vi "U-I.vi"() -> ()   [LabVIEW 2020]
uses:
  <vilib>/Analysis/baseanly.llb/Mean (DBL).vi
  <vilib>/Analysis/NI_AALBase.lvlib
  <vilib>/Analysis/NI_AALPro.lvlib
panel:
  out "数据":dbl[][](array[numeric])
  out "待测电阻值":dbl
  in  "电压上限（V）":dbl
  in  "电压递增步长（V)":dbl
  in  "采集时间间隔":dbl[unit]
  in  "标准电阻值（欧姆）":dbl
  in  "开关":bool
  out "电阻的伏安特性曲线图":cluster{"Y":dbl[], "Y":dbl[]}[](graph)
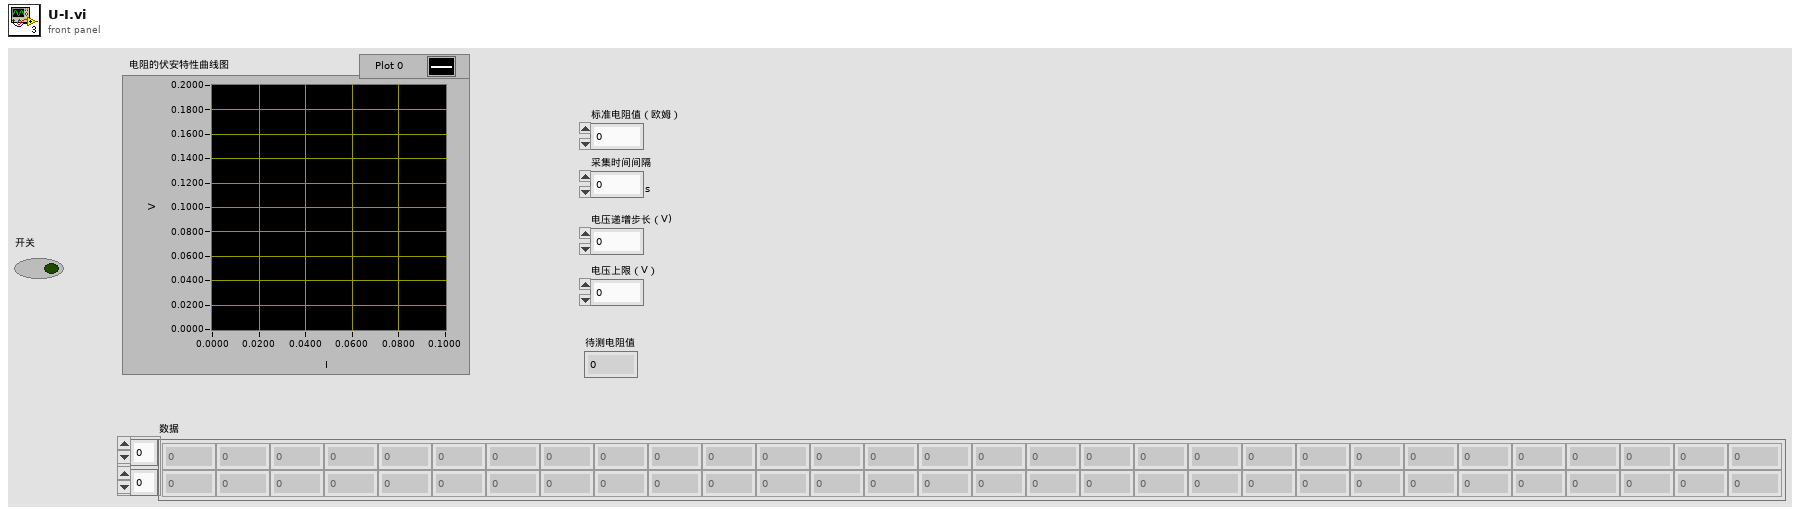
[diagram p1: front panel]
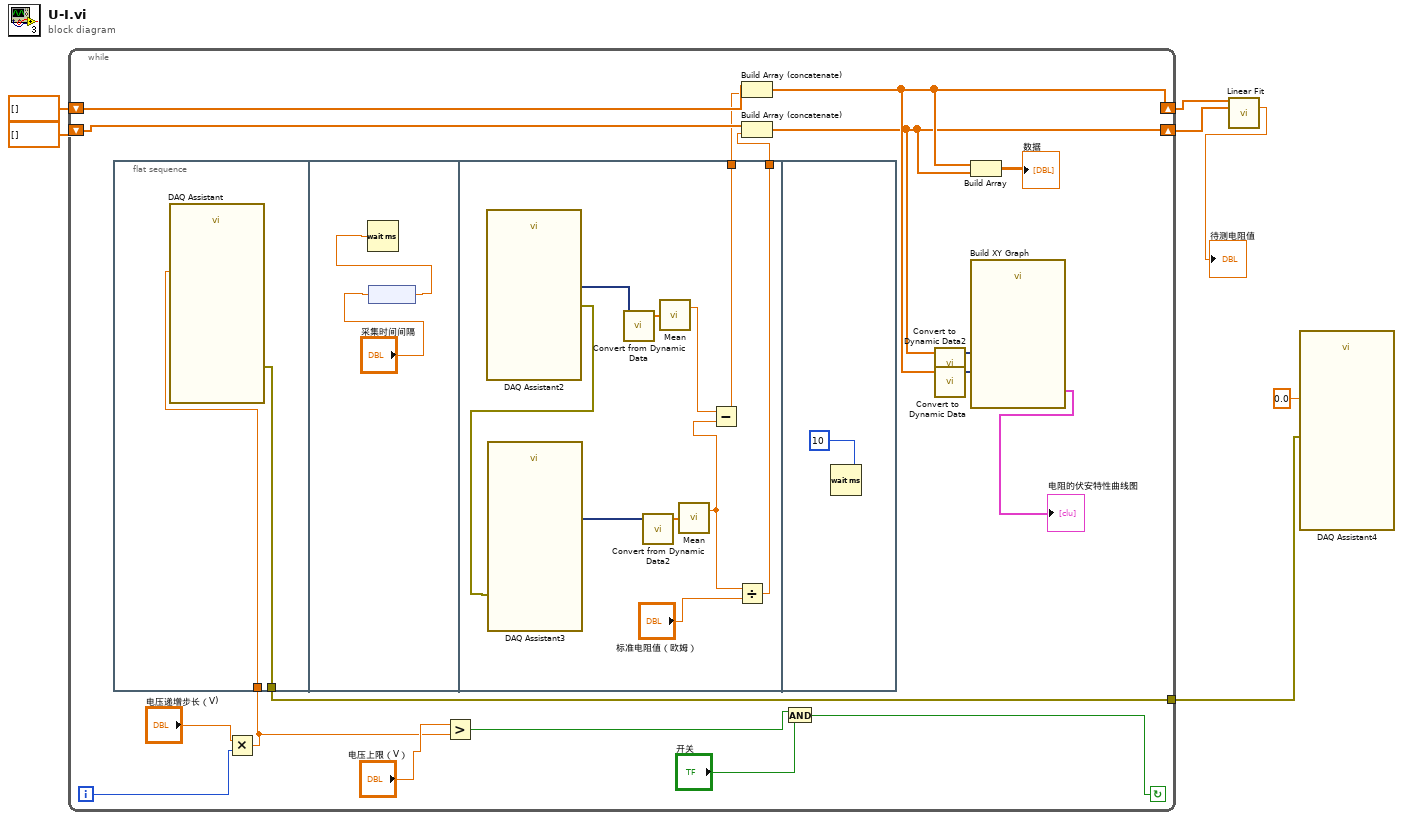
[diagram p0: block diagram]
diagram:
  n1 = while {
    shift-right: [w9] -> w2
    shift-left: dbl[] [] -> [w18]
    shift-right: [w11] -> w1
    shift-left: dbl[] [] -> [w19]
    tunnel: [w14] -> w3
    i -> [w24]
    stop <- w20 continue-if-true
    n2 = flat-sequence {
      tunnel: [w27] -> w14
      tunnel: w12 -> [w26]
      tunnel: [w31] -> w17
      tunnel: [w30] -> w16
      frame #0 {
        n3 = call "DAQ Assistant"("data"=w26) -> ("error out"=w27:errorcluster)  [unwired: 17 in, 1 out]
      }
      frame #1 {
        n4 = node("采集时间间隔") -> (w28:dbl)
        n5 = Wait (ms)(milliseconds to wait=w28) -> ()  [unwired: 1 out]
      }
      frame #2 {
        n6 = call "DAQ Assistant2"() -> ("data"=w38:dynamicdata, "error out"=w39:errorcluster)  [unwired: 17 in, 1 out]
        n7 = call "DAQ Assistant3"("error in"=w39) -> ("data"=w36:dynamicdata)  [unwired: 16 in, 2 out]
        n8 = call "Convert from Dynamic Data"("Dynamic Data Type"=w38) -> ("Array"=w37:dbl[])  [unwired: 3 in]
        n9 = call "Convert from Dynamic Data2"("Dynamic Data Type"=w36) -> ("Array"=w35:dbl[])  [unwired: 3 in]
        n10 = call-poly <vilib>:"Mean.vi"("X"=w37) -> ("mean"=w34:dbl)  [unwired: 1 out]
        n11 = call-poly <vilib>:"Mean.vi"("X"=w35) -> ("mean"=w33:dbl)  [unwired: 1 out]
        n12 = Subtract(x=w34, y=w33) -> (x-y=w31:dbl)
        n13 = Divide(x=w33, y="标准电阻值（欧姆）") -> (x/y=w30:dbl)
      }
      frame #3 {
        n14 = Wait (ms)(milliseconds to wait=u32 10 ("millisecond timer value")) -> ()  [unwired: 1 out]
      }
    }
    n15 = Multiply(x="电压递增步长（V)", y=w24) -> (x*y=w12:dbl)
    n16 = Greater?(x="电压上限（V）", y=w12) -> (0:w22:bool)
    n17 = Build Array (concatenate)(w19, w17) -> (w11:dbl[])
    n18 = Build Array (concatenate)(w18, w16) -> (w9:dbl[])
    n19 = And(x=w22, y="开关") -> (x .and. y?=w20:bool)
    n20 = call "Convert to Dynamic Data2"("Array"=w9) -> ("Dynamic Data Type"=w8:dynamicdata)  [unwired: 3 in]
    n21 = call "Convert to Dynamic Data"("Array"=w11) -> ("Dynamic Data Type"=w10:dynamicdata)  [unwired: 3 in]
    n22 = Build Array(w11, w9) -> (→"数据":dbl[][])
    n23 = call "Build XY Graph"("Y Input"=w10, "X Input"=w8) -> ("XY Graph"=→"电阻的伏安特性曲线图":cluster{"X":dbl[], "Y":dbl[]}[])  [unwired: 8 in, 1 out]
  }
  n24 = call <vilib>:"Linear Fit.vi"("Y"=w1, "X"=w2) -> ("slope"=→"待测电阻值":dbl)  [unwired: 9 in, 4 out]
  n25 = call "DAQ Assistant4"("data"=0.0, "error in"=w3) -> ()  [unwired: 16 in, 2 out]
